vi "H5Tinsert.vi"(0 "error in (no error)":errorcluster, 2 "field_id":i32, 6 "dtype_id":i32, 7 "name":string, 9 "offset":i64) -> (3 "error out":errorcluster, 10 "status":i32)   [LabVIEW 2009]
uses:
  hdf5dll.dll
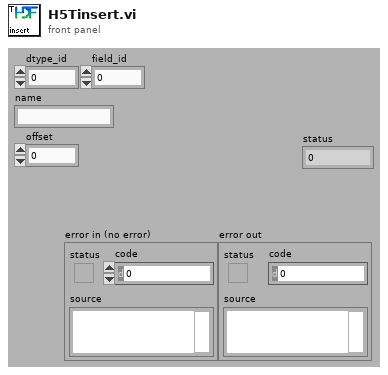
[diagram p1: front panel]
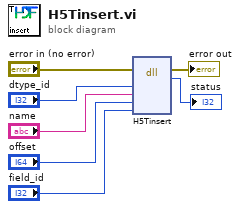
[diagram p0: block diagram]
diagram:
  n1 = dll-call lib="hdf5dll.dll" fn="H5Tinsert"(error in="error in (no error)", "dtype_id"="dtype_id", "name"="name", "offset"="offset", "field_id"="field_id") -> (error out=→"error out":errorcluster, "return type"=→"status":i32)  [unwired: 6 in, 1 out]
